vi "Mappa comandi DCREG.vi"(9 "In marcia":bool=TRUE, 10 "Comandi alimentatori":T1, 11 "output cluster in":T3 {"Alimentatore 1"."Status ref"."RIF 2" scale=0.0..100.0; "Alimentatore 1"."Status ref"."RIF 1" scale=0.0..100.0}) -> (3 "output cluster out":T3 {"Alimentatore 1"."Status ref"."RIF 2" scale=0.0..100.0; "Alimentatore 1"."Status ref"."RIF 1" scale=0.0..100.0})   [LabVIEW 2019]
uses:
  TypeDef/Comandi_Alimentatore.ctl
  Comandi alimentatori.ctl
  cDAQ_PLC Folder/cDAQ/SET SINGLE DO.ctl
  cDAQ_PLC Folder/cDAQ/DO List.ctl
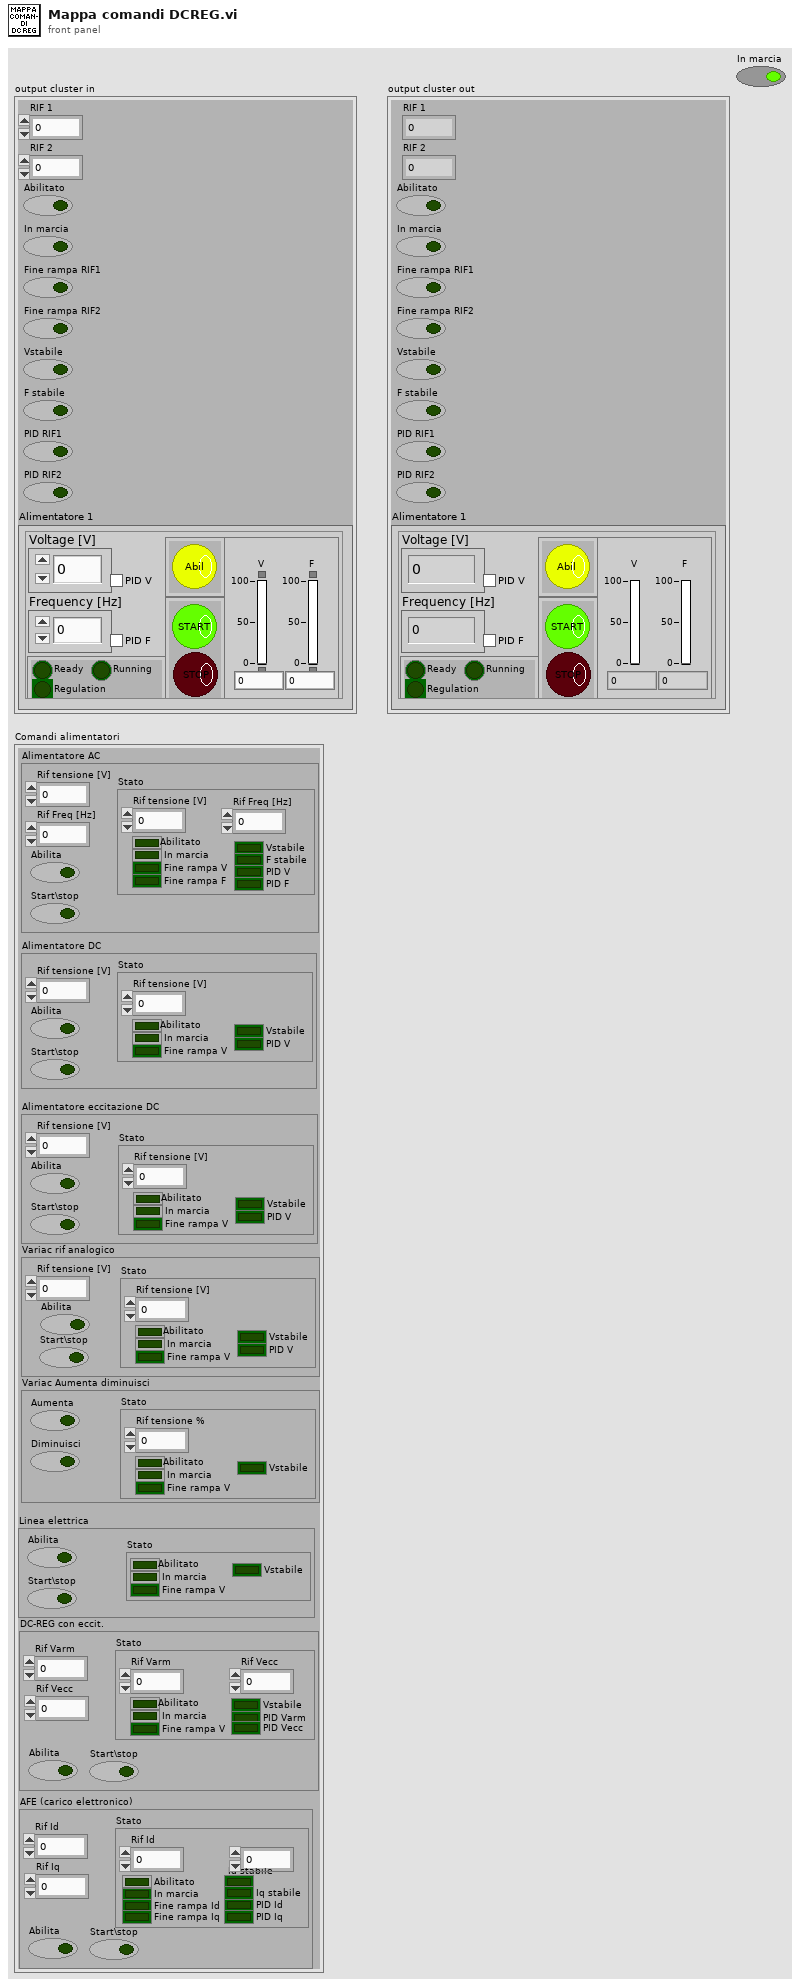
[diagram p1: front panel]
types:
  T1 = typedef "Comandi alimentatori.ctl" = cluster{"Alimentatore AC":cluster{"Rif tensione [V]":dbl, "Rif Freq [Hz]":dbl, "Abilita":bool, "Start\\stop":bool, "Stato":cluster{"Rif tensione [V]":dbl, "Rif Freq [Hz]":dbl, "Abilitato":bool, "In marcia":bool, "Fine rampa V":bool, "Fine rampa F":bool, "Vstabile":bool, "F stabile":bool, "PID V":bool, "PID F":bool}}, "Alimentatore DC":cluster{"Rif tensione [V]":dbl, "Abilita":bool, "Start\\stop":bool, "Stato":cluster{"Rif tensione [V]":dbl, "Abilitato":bool, "In marcia":bool, "Fine rampa V":bool, "Vstabile":bool, "PID V":bool}}, "Variac rif analogico":cluster{"Rif tensione [V]":dbl, "Stato":cluster{"Rif tensione [V]":dbl, "Abilitato":bool, "In marcia":bool, "Fine rampa V":bool, "Vstabile":bool, "PID V":bool}, "Start\\stop":bool, "Abilita":bool}, "Variac Aumenta diminuisci":cluster{"Aumenta":bool, "Diminuisci":bool, "Stato":cluster{"Rif tensione %":dbl, "Abilitato":bool, "In marcia":bool, "Fine rampa V":bool, "Vstabile":bool}}, "Alimentatore eccitazione DC":cluster{"Rif tensione [V]":dbl, "Abilita":bool, "Start\\stop":bool, "Stato":cluster{"Rif tensione [V]":dbl, "Abilitato":bool, "In marcia":bool, "Fine rampa V":bool, "Vstabile":bool, "PID V":bool}}, "Linea elettrica":cluster{"Abilita":bool, "Start\\stop":bool, "Stato":cluster{"Abilitato":bool, "In marcia":bool, "Fine rampa V":bool, "Vstabile":bool}}, "DC-REG con eccit.":cluster{"Rif Varm":dbl, "Abilita":bool, "Start\\stop":bool, "Stato":cluster{"Rif Varm":dbl, "Abilitato":bool, "In marcia":bool, "Fine rampa V":bool, "Vstabile":bool, "PID Varm":bool, "Rif Vecc":dbl, "PID Vecc":bool}, "Rif Vecc":dbl}, "AFE (carico elettronico)":cluster{"Rif Id":dbl, "Abilita":bool, "Start\\stop":bool, "Stato":cluster{"Rif Id":dbl, "Rif Iq":dbl, "Abilitato":bool, "In marcia":bool, "Fine rampa Id":bool, "Fine rampa Iq":bool, "Id stabile":bool, "Iq stabile":bool, "PID Id":bool, "PID Iq":bool}, "Rif Iq":dbl}}
  T2 = typedef "Comandi_Alimentatore.ctl" = cluster{"RIF 1":dbl, "RIF 2":dbl, "Status":cluster{"Ready":bool, "Running":bool, "Regulation":bool}, "Start\\stop":cluster{"Start":bool, "Stop":bool}, "PID RIF1":bool, "PID RIF2":bool, "Status ref":cluster{"RIF 1":dbl, "RIF 2":dbl}, "Abilita":cluster{"Abilita":bool}}
  T3 = cluster{"RIF 1":dbl, "RIF 2":dbl, "Abilitato":bool, "In marcia":bool, "Fine rampa RIF1":bool, "Fine rampa RIF2":bool, "Vstabile":bool, "F stabile":bool, "PID RIF1":bool, "PID RIF2":bool, "Alimentatore 1":T2}
  T4 = typedef "SET SINGLE DO.ctl" = cluster{"DO":T5, "Value":bool}
  T5 = typedef "DO List.ctl" = enum16{"OFF: ALL DO", "*ABILITA freno 1", "*ABILITA freno 2", "*ABILITA freno 3", "*START freno 1", "*START freno 2", "*START freno 3", "*STOP freno 1", "*STOP freno 3", "*STOP freno 2", "*Senso rot freno 1", "*Senso rot freno 2", "*Senso rot freno 3", "*Ctrl velocità freno 1", "*Ctrl velocità freno 2", "*Ctrl velocità freno 3", "*Ctrl coppia freno 1", "*Ctrl coppia freno 2", "*Ctrl coppia freno 3", "*ABILITA alimentatore 1", "*ABILITA alimentatore 2", "*ABILITA alimentatore 3", "*ABILITA alimentatore 4", "*START alimentatore 1", "*START alimentatore 2", "*START alimentatore 3", "*START alimentatore 4", "*STOP alimentatore 1", "*STOP alimentatore 2", "*STOP alimentatore 3", "*STOP alimentatore 4", "SENSO ROT alimentatore 1", "SENSO ROT alimentatore 2", "Abilita LEM 1000A", "Abilita LEM 300A", "Abilita sensori EXT WT", "B1 Seleziona linea 1", "B1 Seleziona linea 2", "B1 Seleziona linea 3", "B1 Seleziona linea 4", "B1 Seleziona linea 5", "B2 Seleziona linea 1", "B2 Seleziona linea 2", "B2 Seleziona linea 3", "B2 Seleziona linea 4", "B2 Seleziona linea 5", "*Reset allarmi", "*Start potenza AC", "*Stop potenza AC", "*Start potenza DC", "*Stop potenza DC", "*Start potenza DC eccit", "*Stop pontenza DC eccit", "Bypass res meter", "2nd canale res meter", "Enable res meter", "*Abilit teler ramo WT", "*Abil teler ramo princ Resit", "*Abil teler ramo 1 Resist", "*Abil teler ramo 2 Resist", "*Abil teler ramo 3 Resist", "*Abil cortocirc avvolgim", "*Controllo torsiometro B1", "*Controllo Torsiom B2", "*Scala torsiometro B1", "*Scala torsiometro B2", "*Collaudo in corso", "*Allarme presente", "Abilitazione elettroserratura", "Exit", "*Abilita collaudo", "*Abilita potenza trifase", "*Abilita potenza monofase", "*Abilita potenza DC", "*Abilita potenza DC eccit", "*Disabilita teleruttori potenza", "Set teleruttori prova a freddo", "Prova a freddo monofase", "Watchdog", "Forza DO PLC 3", "Forza DO PLC 2", "Forza DO PLC 1", "Forza DO cDAQ", "Scala 2000(T) 200(F) res meter", "Seleziona banco 1", "Seleziona banco 2", "Comando azionam in blocco", "Comando azionam reset", "Sensibilità freno 16 32 nm", "Reset Allarmi", "Carico res - Ramo 1", "Carico res - Ramo 2", "Carico res - Ramo 3", "Carico res - Ramo 4", "Carico res - Ramo 5", "Carico res - Ramo 6", "Carico res - Ramo 7", "Carico res - Ramo 8", "Carico res - Ramo 9", "Carico res - Ramo 10", "Carico res - Ramo 11", "Carico res - Start ventilatore", "Carico res - Stop ventilatore", "Abilita potenza solo freno", "Abilita AFE + freno trasc", "Abilita potenza carico resistivo", "Chiudi potenza AFE", "Apri potenza AFE", "Start AFE", "Config Banco2 TDE", "Misura diretto WT", "Ripristina centralina protezioni", "Abilita Scrittura Dati Keb", "Bench Selection(0-B1,1-B2)", "Select current mode", "Select torque mode", "Select speed mode", "Extenal alarm", "Enable Extenal program ", "Start ", "Stop", "Enable force mode", "Abilita linea 125 A", "Abilita linea 63 A", "Abilita linea 16 A", "Aum Tensione Variac", "Dim Tesnione Variac", "Abilita Ellecto Stractura", "Riprinto Emergenxe ", "Abilita Collaudo", "Disabilita Collaudo", "Abilita Ingresso Variac", "Abilita Uscita Variac", "Abilita ventilatore Variac"}
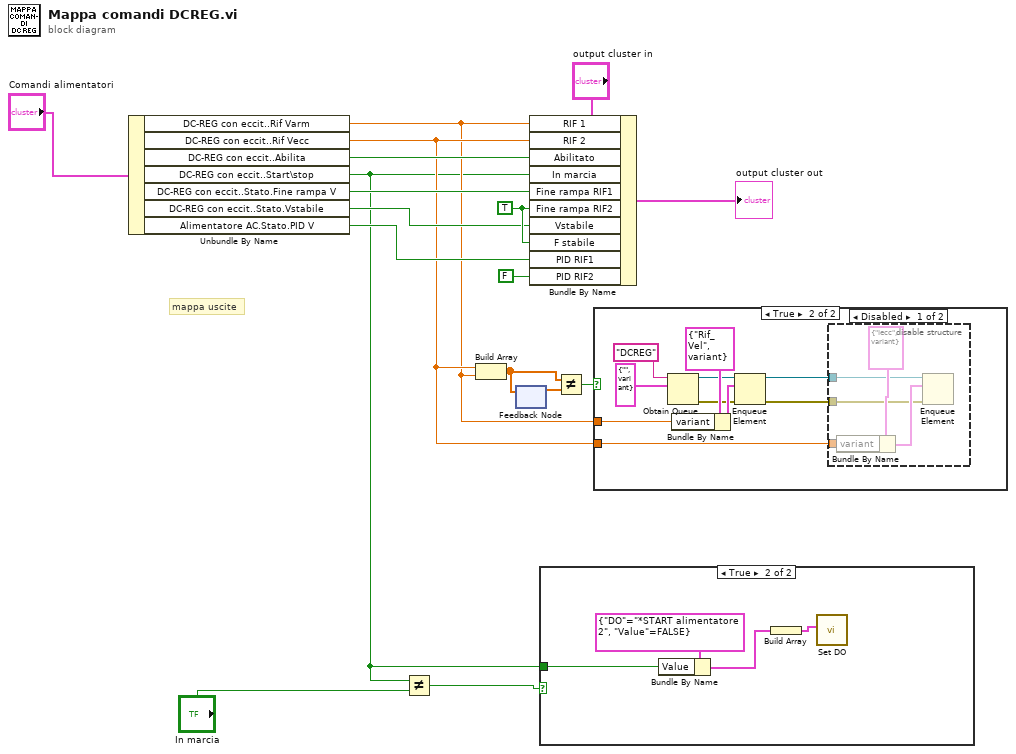
[diagram p0: block diagram]
diagram:
  w16 = TRUE ("Fine rampa RIF2")
  # "mappa uscite"
  n1 = Unbundle By Name("Comandi alimentatori") -> ("DC-REG con eccit..Rif Varm"=w7:dbl, "DC-REG con eccit..Rif Vecc"=w8:dbl, "DC-REG con eccit..Abilita"=w15:bool, "DC-REG con eccit..Start\\stop"=w3:bool, "DC-REG con eccit..Stato.Fine rampa V"=w11:bool, "DC-REG con eccit..Stato.Vstabile"=w12:bool, "Alimentatore AC.Stato.PID V"=w13:bool)
  n2 = Not Equal?(x=w3, y="In marcia") -> (x != y?=w1:bool)
  n3 = Build Array(w8, w7) -> (w6:dbl[])
  n4 = feedback-in #1(w6) -> ()
  n5 = feedback #1() -> (w5:dbl[])  [unwired: 1 in]
  n6 = Bundle By Name(cluster="output cluster in", "RIF 1"=w7, "RIF 2"=w8, "Abilitato"=w15, "In marcia"=w3, "Fine rampa RIF1"=w11, "Fine rampa RIF2"=w16, "Vstabile"=w12, "F stabile"=w16, "PID RIF1"=w13, "PID RIF2"=FALSE) -> (→"output cluster out":T3)
  n7 = case shown="True" w1 {
    tunnel: w3 -> [_ w18]
    frame False {
    }
    frame True {
      n8 = Bundle By Name(cluster=T4 {"DO"=enum."*START alimentatore 2", "Value"=FALSE} ("Cluster SET DO"), "Value"=w18) -> (w20:T4)
      n9 = Build Array(w20) -> (w21:T4[])
      n10 = call "Set DO.vi"("Cluster SET DO"=w21) -> ()  [unwired: 10 in, 1 out]
    }
  }
  n11 = Not Equal?(x=w6, y=w5) -> (x != y?=w4:bool)
  n12 = case shown="True" w4 {
    tunnel: w8 -> [_ w23]
    tunnel: w7 -> [_ w22]
    frame False {
    }
    frame True {
      n13 = Obtain Queue(name (unnamed)="DCREG", element data type=cluster{"String":string, "variant":variant} {"String"="", "variant"=variant} ("element")) -> (queue out=w27:refnum<queue>, error out=w25:errorcluster)  [unwired: 3 in, 1 out]
      n14 = Bundle By Name(cluster=cluster{"String":string, "variant":variant} {"String"="Rif_Vel", "variant"=variant} ("element"), "variant"=w22) -> (w29:cluster{"String":string, "variant":variant})
      n15 = Enqueue Element(queue=w27, element=w29, error in (no error)=w25) -> (queue out=w31:refnum<queue>, error out=w30:errorcluster)  [unwired: 1 in, 1 out]
      n16 = disable-structure shown="Disabled" {
        disable-tunnel: w31 -> [w34 _]
        disable-tunnel: w30 -> [w33 _]
        disable-tunnel: w23 -> [w32 _]
        frame Disabled {
          n17 = Bundle By Name(cluster=cluster{"String":string, "variant":variant} {"String"="Iecc", "variant"=variant} ("element"), "variant"=w32) -> (w36:cluster{"String":string, "variant":variant})
          n18 = Enqueue Element(queue=w34, element=w36, error in (no error)=w33) -> ()  [unwired: 1 in, 3 out]
        }
        frame Enabled {
        }
      }
    }
  }
